vi "Demo.vi"() -> ()   [LabVIEW 2020, in "UDS.lvclass"]
uses:
  UDS.lvclass
  <vilib>/Automotive Diagnostic Command Set/Diagnostic Transport.llb/Property ID.ctl
  <vilib>/addons/_AddQ/G#Object/G#Object.lvclass
  <vilib>/addons/Automotive Diagnostic Command Set/NI_Automotive Diagnostic Command Set.lvlib
panel:
  out "DataIdentify":string
  out "Clear DTC":bool
  out "DID":u8[](array[numeric]) format="%.0x"
  out "OK":bool
  out "# of objects killed":i32
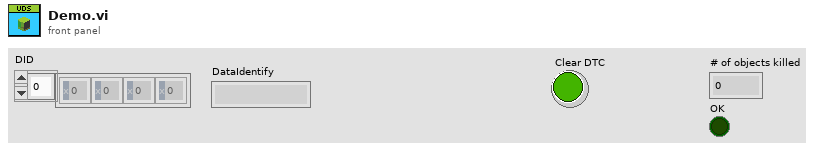
[diagram p1: front panel]
types:
  T1 = typedef "NI_Automotive Diagnostic Command Set.lvlib/Property ID.ctl" = enum16{"Timeout Diag Command", "Timeout FC (Bs)", "Timeout CF (Cr)", "Receive Block Size (BS)", "Wait Time CF (STmin)", "Max Wait Frames (N_WFTmax)", "Wait Frames to Send (N_WAIT)", "Time between Waits (T_W)", "Fill CAN Frames", "Fill Byte", "Invalid Response as Error", "Max RspPending Count", "VWTP Command Timeout", "STmin", "P2min", "Termination", "Timeout RspPending", "LIN Sleep", "Actual CAN IO Mode", "Response Plausibility Check", "Session-based Properties"}
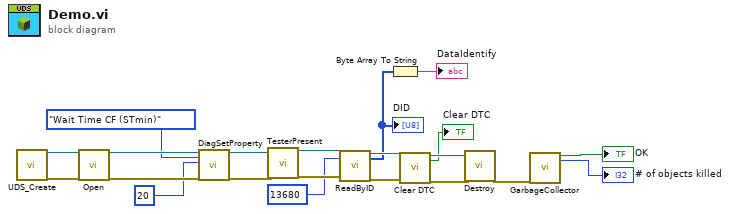
[diagram p0: block diagram]
diagram:
  n1 = call "UDS_Create.vi"() -> ("reference out"=w21:refnum<class "UDS.lvclass">, "error out"=w20:errorcluster)  [unwired: 18 in]
  n2 = call-dynamic "Open.vi"("reference in"=w21, "error in (no error)"=w20) -> ("reference out"=w19:refnum<class "UDS.lvclass">, "error out"=w18:errorcluster)  [unwired: 16 in]
  n3 = call-dynamic "DiagSetProperty.vi"("reference in"=w19, "property ID"=Property_ID."Wait Time CF (STmin)", "property value"=u32 20, "error in (no error)"=w18) -> ("reference out"=w17:refnum<class "UDS.lvclass">, "error out"=w16:errorcluster)  [unwired: 14 in]
  n4 = call-dynamic "TesterPresent.vi"("reference in"=w17, "error in (no error)"=w16) -> ("reference out"=w15:refnum<class "UDS.lvclass">, "error out"=w14:errorcluster)  [unwired: 16 in]
  n5 = call-dynamic "ReadByID.vi"("reference in"=w15, "ID"=u16 13680, "error in (no error)"=w14) -> ("reference out"=w13:refnum<class "UDS.lvclass">, "DID"=w2:u8[], "error out"=w12:errorcluster)  [unwired: 14 in]
  "DID" <- w2
  n6 = Byte Array To String(unsigned byte array=w2) -> (string=→"DataIdentify":string)
  n7 = call-dynamic "Clear DTC.vi"("reference in"=w13, "error in (no error)"=w12) -> ("reference out"=w11:refnum<class "UDS.lvclass">, "Clear DTC"=→"Clear DTC":bool, "error out"=w10:errorcluster)  [unwired: 15 in]
  n8 = call-dynamic "Destroy.vi"("reference in"=w11, "error in (no error)"=w10) -> ("error out"=w7:errorcluster)  [unwired: 16 in, 1 out]
  n9 = call <vilib>:"GarbageCollector.vi"("error in (no error)"=w7) -> ("OK"=→"OK":bool, "# of objects killed"=→"# of objects killed":i32)  [unwired: 16 in, 1 out]
